vi "H5D_write_cluster.vi"(4 "Dust Array":T1[](array[typedef]) {"File Location" items=["Currently Writing"=-3, "Labview Files"=-2, "Mars Data Processing Factility"=-1, "Local Cache "=0, "Old Storage"=1, "Storage"=2]; "Estimate Source" items=["Any Source."=-2, "No Shot"=-1, "Basic Labview Estimate"=0, "IDL Estimate From Andrew"=1, "IDL Estimate From Tobin"=2, "Old Metadata"=3]}, 5 "name":string, 6 "error in (no error)":errorcluster, 7 "overwrite?":bool, 8 "preserve attribs?":bool, 9 "ref":i32) -> (0 "error out":errorcluster, 3 "ref out":i32)   [LabVIEW 2012]
doc: "Creates a dataset with the specified name from the data variant. Arrays are turned into dataspaces and types converted.\n\nIf the dataset exists and both \"overwrite\" and \"preserve attribs\" are specified, then the attributes of the dataset are kept intact."
uses:
  Public API/Query_Dust_Event.ctl
  Estimate_source.ctl
  File_location.ctl
  <vilib>/addons/h5labview/H5_errcode.vi
  <vilib>/Utility/error.llb/Error Cluster From Error Code.vi
  <vilib>/addons/h5labview/H5Base.lvlib
  <vilib>/addons/_h5labview_internal_deps/hdf5dll.dll
  <vilib>/addons/h5labview/H5Attrib.lvlib
panel:
  # "Dust Event"
  # "h5labview :: H5D"
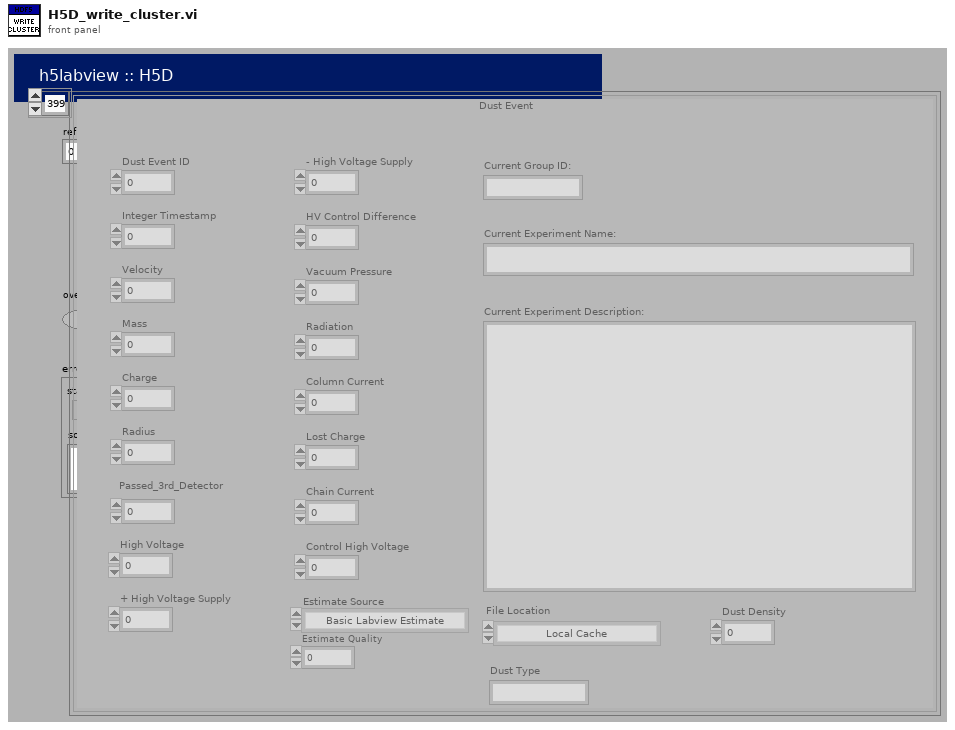
[diagram p1: front panel]
types:
  T1 = typedef "Query_Dust_Event.ctl" = cluster{"Dust Event ID":i64, "Integer Timestamp":i64, "Velocity":sgl, "Mass":sgl, "Charge":sgl, "Radius":sgl, "Passed_3rd_Detector":i8, "High Voltage":sgl, "+ High Voltage Supply":sgl, "- High Voltage Supply":sgl, "HV Control Difference":sgl, "Vacuum Pressure":sgl, "Radiation":sgl, "Column Current":sgl, "Lost Charge":sgl, "Chain Current":sgl, "Control High Voltage":sgl, "Current Group ID:":string, "Current Experiment Name:":string, "Current Experiment Description:":string, "Estimate Source":T2, "Estimate Quality":sgl, "File Location":T3, "Dust Type":string, "Dust Density":sgl}
  T2 = typedef "Estimate_source.ctl" = i8
  T3 = typedef "File_location.ctl" = i8
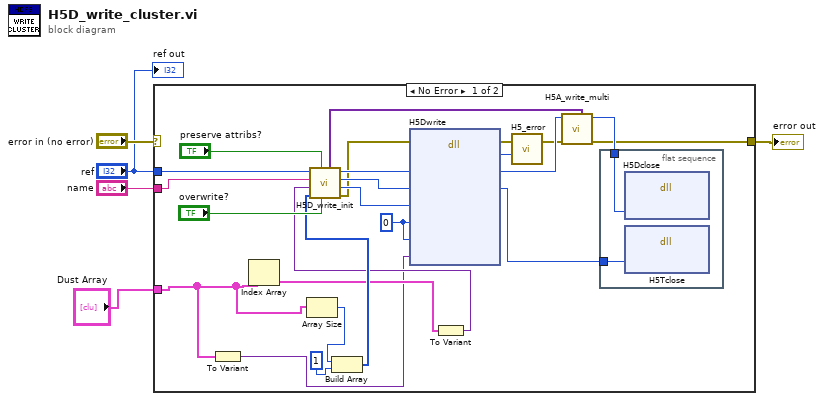
[diagram p0: block diagram]
diagram:
  n1 = case shown="No Error" "error in (no error)" {
    selector: "error in (no error)" -> [_ w32]
    tunnel: [w13 w32] -> w2
    tunnel: "ref" -> [w21 _]
    tunnel: "name" -> [w20 _]
    tunnel: "Dust Array" -> [w7 _]
    frame No Error {
      w15 = 0 ("file_space_id")
      n2 = To Variant(anything=w7) -> (Variant=w6:variant)
      n3 = Index Array(array=w7) -> (element=w9:T1)  [unwired: 1 in]
      n4 = Array Size(array=w7) -> (size(s)=w11:i32)
      n5 = Build Array(w11, 1 ("element")) -> (w12:i32[])
      n6 = To Variant(anything=w9) -> (Variant=w8:variant)
      n7 = call <vilib>:"H5D_write_init.vi"("overwrite?"="overwrite?", "preserve attribs?"="preserve attribs?", "dims"=w12, "type"=w8, "name"=w20, "ref"=w21) -> ("error out"=w14:errorcluster, "space"=w16:i32, "dtype"=w17:i32, "ds_id"=w25:i32, "attribs"=w24:variant[])
      n8 = dll-call lib="C:/Program Files (x86)/National Instruments/LabVIEW 2012/vi.lib/addons/_h5labview_internal_deps/hdf5dll.dll" fn="H5Dwrite" ("hdf5_call")(error in=w14, "ds_id"=w25, "mem_type"=w17, "mem_space"=w16, "file_space_id"=w15, "xfer_plist_id"=w15, "buffer"=w6) -> (error out=w27:errorcluster, "return type"=w26:i32, "ds_id"=w29:i32, "mem_type"=w28:i32)  [unwired: 6 in, 1 out]
      n9 = call <vilib>:"H5_error.vi"("retval"=w26, "error in (no error)"=w27) -> ("error out"=w23:errorcluster)  [unwired: 1 out]
      n10 = call <vilib>:"H5A_write_multi.vi"("attribs"=w24, "error in (no error)"=w23, "ref"=w29) -> ("error out"=w13:errorcluster, "ref out"=w18:i32)  [unwired: 5 in]
      n11 = flat-sequence {
        tunnel: w28 -> [w31]
        tunnel: w18 -> [w30]
        frame #0 {
          n12 = dll-call lib="C:/Program Files (x86)/National Instruments/LabVIEW 2012/vi.lib/addons/_h5labview_internal_deps/hdf5dll.dll" fn="H5Dclose" ("hdf5_call")("ds_id"=w30) -> ()  [unwired: 5 in, 2 out]
          n13 = dll-call lib="C:/Program Files (x86)/National Instruments/LabVIEW 2012/vi.lib/addons/_h5labview_internal_deps/hdf5dll.dll" fn="H5Tclose" ("hdf5_call")("t_id"=w31) -> ()  [unwired: 5 in, 2 out]
        }
      }
    }
    frame Error {
    }
  }
  "error out" <- w2
  "ref out" <- "ref"
